vi "array_problem_3.vi"() -> ()   [LabVIEW 2020]
panel:
  in  "Delay":dbl
  out "Boolean Rotated Array":bool[](array[boolean])
  out "Boolean Array":bool[](array[boolean])
  out "Rotated Array":dbl[](array[numeric])
  in  "Array":dbl[](array[numeric])
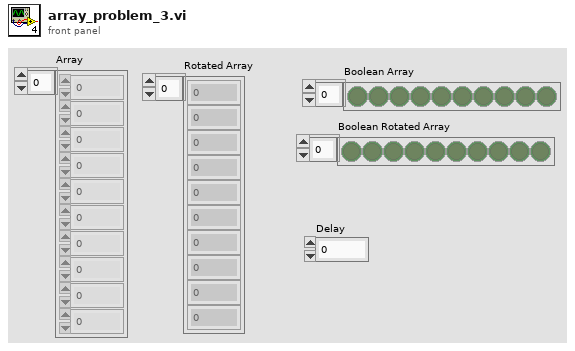
[diagram p1: front panel]
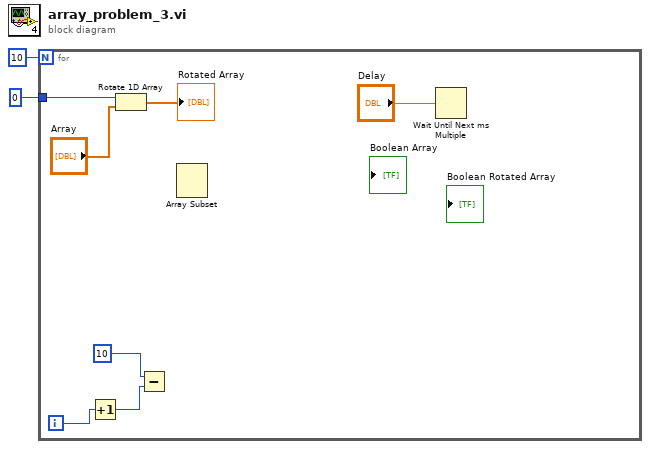
[diagram p0: block diagram]
diagram:
  n1 = for {
    N: 10 -> [_]
    tunnel: 0 -> [w4]
    i -> [w8]
    n2 = Increment(x=w8) -> (x+1=w6:i32)
    n3 = Rotate 1D Array(1:"Array", 2:w4) -> (0:→"Rotated Array":dbl[])
    n4 = Subtract(x=10, y=w6) -> ()  [unwired: 1 out]
    n5 = Array Subset() -> ()  [unwired: 3 in, 1 out]
    n6 = Wait Until Next ms Multiple(millisecond multiple="Delay") -> ()  [unwired: 1 out]
  }
